vi "Scenario Get Scenario.vi"(8 "error in (no error)":errorcluster, 9 "Retrieve Conditions? (t)":bool=TRUE, 10 "Query":string, 11 "Connection Refnum":T4) -> (0 "error out":errorcluster, 2 "Scenarios":T1[](array[typedef]), 3 "Connection Refnum":T4, 4 "Data Present?":bool)   [LabVIEW 2011]
uses:
  SI.LIB/ODBC/SQL Controls/Connection Refnum.ctl
  Scenario Record.ctl
  Conditions/Condition Record.ctl
  Conditions/Condition Operators.ctl
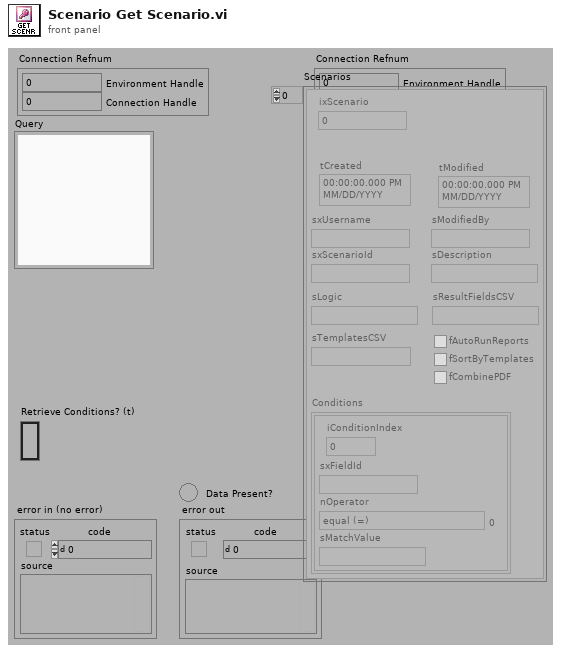
[diagram p1: front panel]
types:
  T1 = typedef "Scenario Record.ctl" = cluster{"ixScenario":i32, "tCreated":timestamp, "tModified":timestamp, "sxUsername":string, "sModifiedBy":string, "sxScenarioId":string, "sDescription":string, "sLogic":string, "sResultFieldsCSV":string, "sTemplatesCSV":string, "fAutoRunReports":bool, "fSortByTemplates":bool, "fCombinePDF":bool, "Conditions":T2[]}
  T2 = typedef "Condition Record.ctl" = cluster{"iConditionIndex":i32, "sxFieldId":string, "nOperator":T3, "sMatchValue":string}
  T3 = typedef "Condition Operators.ctl" = enum16{"equal (=)", "not equal (\\u2260)", "less than (<)", "less than or equal (\\u2264)", "greater than (>)", "greater than or equal (\\u2265)", "contains", "does not contain"}
  T4 = typedef "Connection Refnum.ctl" = cluster{"Environment Handle":i32, "Connection Handle":i32}
  T5 = typedef "Statement Refnum.ctl" = cluster{"Statement Handle":i32, "Parameter Number":u16}
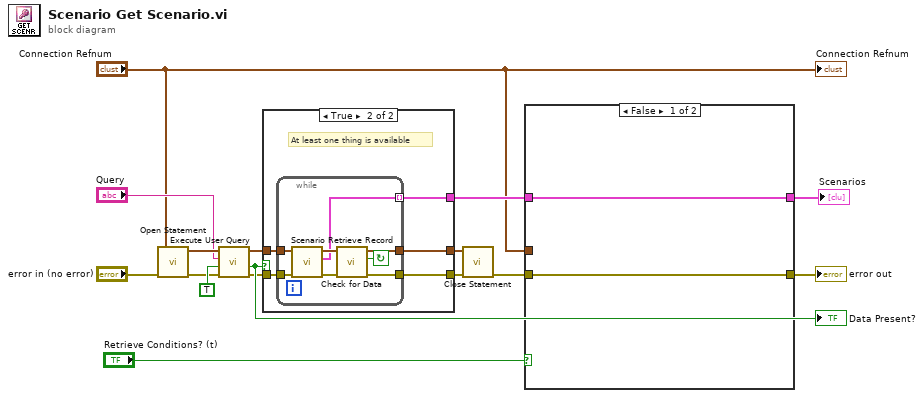
[diagram p0: block diagram]
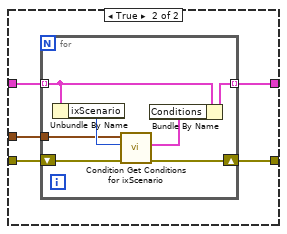
[diagram p2: hidden frame]
diagram:
  n1 = call "Open Statement.vi"("error in (no error)"="error in (no error)", "Connection Refnum"="Connection Refnum") -> ("error out"=w11:errorcluster, "Statement Refnum"=w12:T5)  [unwired: 4 out]
  n2 = call "Execute User Query.vi"("error in (no error)"=w11, "Return Data? (f)"=TRUE, "User Query"="Query", "Statement Refnum"=w12) -> ("error out"=w15:errorcluster, "Data Present?"=w16:bool, "Statement Refnum"=w14:T5)  [unwired: 1 out]
  "Data Present?" <- w16
  n3 = case shown="True" w16 {
    tunnel: w15 -> [w17 w22]
    tunnel: w14 -> [w18 w23]
    tunnel: [w17 w20] -> w10
    tunnel: [w18 w21] -> w9
    tunnel: [_ w19] -> w4
    frame False {
      # "Query Returned no matching fields."
    }
    frame True {
      # "At least one thing is available"
      n4 = while {
        tunnel: w23 -> [w30]
        tunnel: w22 -> [w29]
        tunnel: [w27] -> w21
        tunnel: [w25] -> w20
        tunnel: [w24] -> w19 mode=indexing
        stop <- w31 continue-if-true
        n5 = call "Scenario Retrieve Record.vi"("error in (no error)"=w29, "Statement Refnum"=w30) -> ("error out"=w26:errorcluster, "Scenario"=w24:T1, "Statement Refnum"=w28:T5)  [unwired: 7 out]
        n6 = call "Check for Data.vi"("error in (no error)"=w26, "Statement Refnum"=w28) -> ("error out"=w25:errorcluster, "Data Present?"=w31:bool, "Statement Refnum"=w27:T5)  [unwired: 3 out]
      }
    }
  }
  n7 = call "Close Statement.vi"("error in (no error)"=w10, "Statement Refnum"=w9) -> ("error out"=w6:errorcluster)  [unwired: 5 out]
  n8 = case shown="False" "Retrieve Conditions? (t)" {
    tunnel: w6 -> [w32 w38]
    tunnel: [w32 w37] -> w5
    tunnel: w4 -> [w33 w36]
    tunnel: "Connection Refnum" -> [_ w35]
    tunnel: [w33 w34] -> w2
    frame False {
    }
    frame True {
      n9 = for {
        shift-right: [w44] -> w37
        shift-left: w38 -> [w45]
        tunnel: w36 -> [w41] mode=indexing
        tunnel: w35 -> [w42]
        tunnel: [w39] -> w34 mode=indexing
        n10 = Unbundle By Name(w41) -> ("ixScenario"=w43:i32)
        n11 = call "Condition Get Conditions for ixScenario.vi"("error in (no error)"=w45, "ixScenario (0)"=w43, "Connection Refnum"=w42) -> ("error out"=w44:errorcluster, "Conditions"=w40:T2[])  [unwired: 7 out]
        n12 = Bundle By Name(cluster=w41, "Conditions"=w40) -> (w39:T1)
      }
    }
  }
  "error out" <- w5
  "Scenarios" <- w2
  "Connection Refnum" <- "Connection Refnum"
